vi "Write App Mgr.vi"(8 "error in (no error)":errorcluster, 10 "App Mgr":refnum<k7>, 11 "Main in":refnum<class "Main.lvclass">) -> (0 "error out":errorcluster, 3 "Main out":refnum<class "Main.lvclass">)   [LabVIEW 2023, in "GUI.lvlib" / "Main.lvlib" / "Main.lvclass"]
uses:
  Main.lvclass
  Main.lvclass/Main.ctl
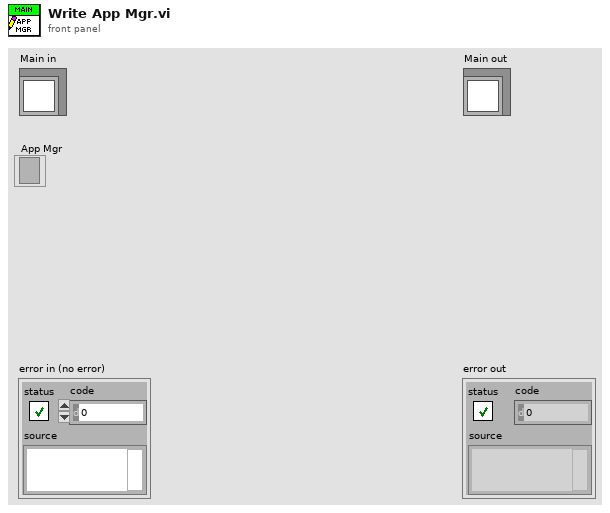
[diagram p1: front panel]
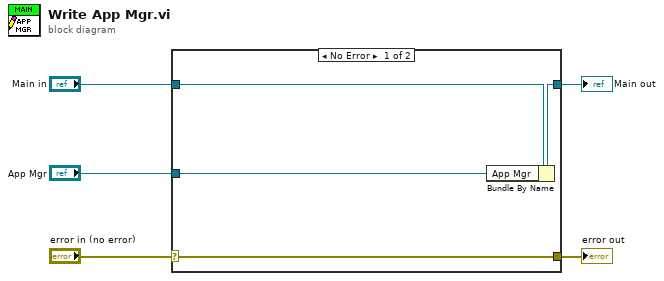
[diagram p0: block diagram]
diagram:
  n1 = case shown="No Error" "error in (no error)" {
    selector: "error in (no error)" -> [w9 w10]
    tunnel: [w9 w10] -> w4
    tunnel: [w7 w11] -> w2
    tunnel: "Main in" -> [w8 w11]
    tunnel: "App Mgr" -> [w6 _]
    frame No Error {
      n2 = Bundle By Name(cluster=w8, "App Mgr"=w6) -> (w7:refnum<class "Main.lvclass">)
    }
    frame Error {
    }
  }
  "error out" <- w4
  "Main out" <- w2
